vi "Read PluginPathArray.vi"(8 "error in (no error)":errorcluster, 11 "TestBase in":refnum<class "TestBase.lvclass">) -> (0 "error out":errorcluster, 2 "PluginPathArray":path[][](array[path]), 3 "TestBase out":refnum<class "TestBase.lvclass">)   [LabVIEW 2014, in "TestBase.lvclass"]
uses:
  TestBase.lvclass
  TestBase.lvclass/TestBase.ctl
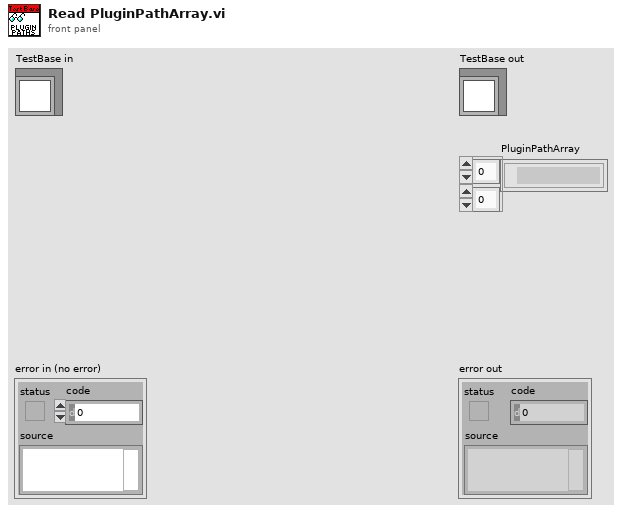
[diagram p1: front panel]
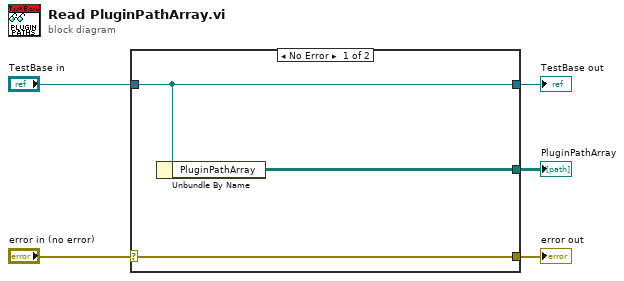
[diagram p0: block diagram]
diagram:
  n1 = case shown="No Error" "error in (no error)" {
    selector: "error in (no error)" -> [w8 w9]
    tunnel: [w8 w9] -> w4
    tunnel: [w7 w10] -> w2
    tunnel: "TestBase in" -> [w7 w10]
    tunnel: [w6 _] -> w1
    frame No Error {
      n2 = Unbundle By Name(w7) -> ("PluginPathArray"=w6:path[][])
    }
    frame Error {
    }
  }
  "error out" <- w4
  "TestBase out" <- w2
  "PluginPathArray" <- w1
